vi "LoadDataSPC130.vi"(5 "Path":refnum<vi>) -> (0 "gap photons":u32, 1 "invalid photons":u32, 2 "total":u32)   [LabVIEW 2009]
panel:
  out "% done":dbl(slide) scale=0.0..100.0
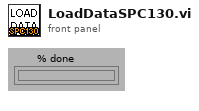
[diagram p1: front panel]
types:
  T1 = enum16{"Display", "change", "Get", "Set", "Set Ken"}
  T2 = typedef "FIFOSettings_BH.ctt" = cluster{"Measurement":cluster{"Binning (ms)":sgl, "External Trigger Condition":u16, "Stop Condition:":u16, "Stop Count":dbl, "Buffer Size (Photons)":u16, "No of Channels":u16, "Ext Latch Delay":i16}, "ADC":cluster{"Module":u16, "ADC Resolution":i32, "Dither Range":i16, "Count Increment":i16, "Macro Time Clock":i16}, "SYNC":cluster{"SYNC ZC Level (mV)":sgl, "SYNC Freq Divider":i16, "SYNC Holdoff (ns)":sgl, "SYNC Threshold (mV)":sgl}, "TAC":cluster{"TAC Range (ns)":sgl, "TAC Gain":i16, "TAC Offset (%)":sgl, "TAC Limit Low (%)":sgl, "TAC Limit High (%)":sgl}, "CFD":cluster{"CFD Limit Low (mV)":sgl, "CFD Limit High (mV)":sgl, "CFD ZC Level (mV)":sgl, "CFD Holdoff (ns)":sgl}}
  T3 = cluster{"router channels":u8[], "macro times":dbl[], "micro times":u16[], "invalid times":dbl[], "gap times":dbl[]}
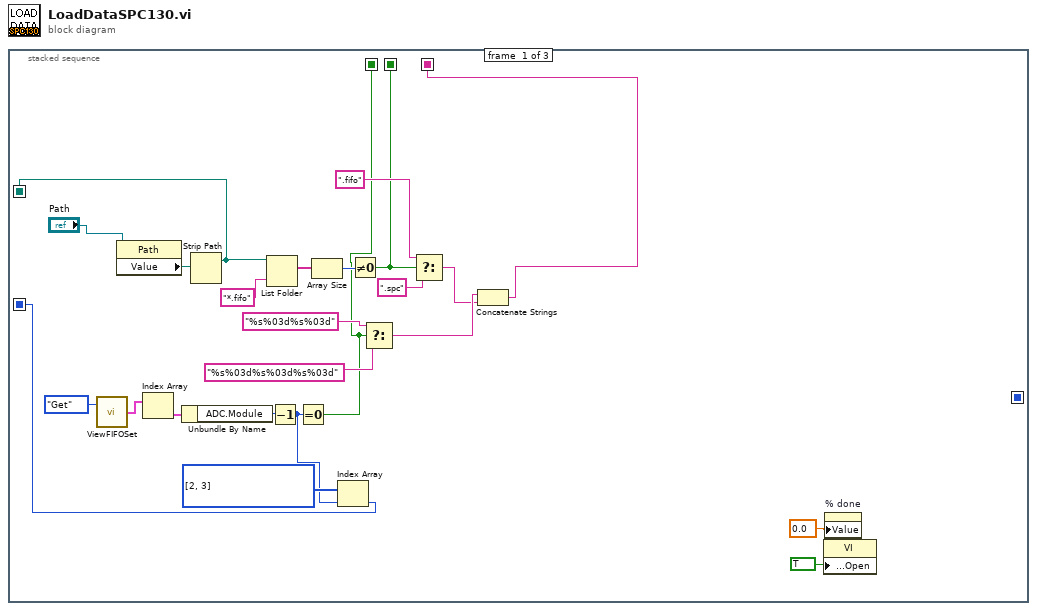
[diagram p0: block diagram]
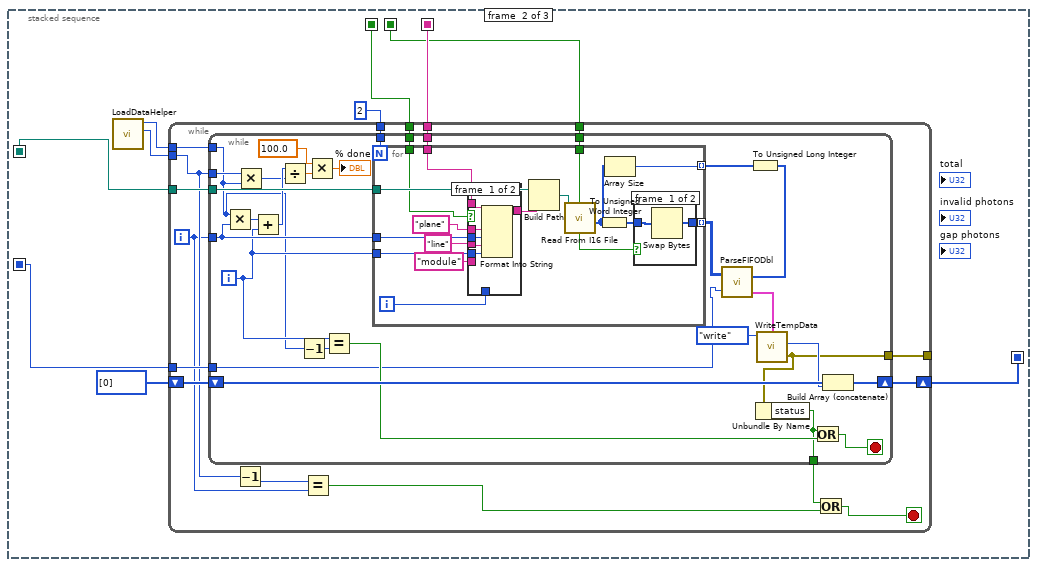
[diagram p2: hidden frame]
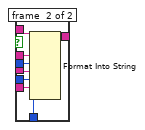
[diagram p3: hidden frame]
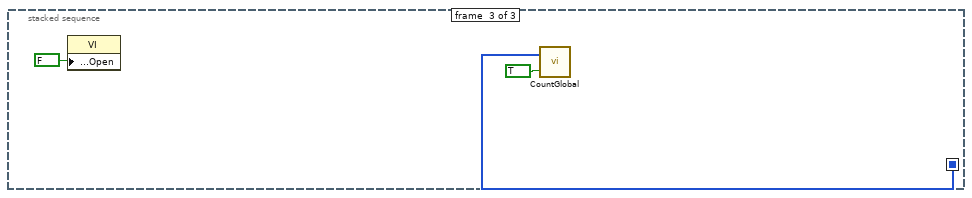
[diagram p5: hidden frame]
diagram:
  n1 = stacked-sequence {
    seq-local: [_ w33 _] -> [_ _ w115]
    seq-local: [w16 _ _] -> [_ w29 _]
    seq-local: [w15 _ _] -> [_ w25 _]
    seq-local: [w6 _ _] -> [_ w28 _]
    seq-local: [w2 _ _] -> [_ w27 _]
    seq-local: [w1 _ _] -> [_ w26 _]
    frame #0 {
      w4 = u16[] [2, 3] items=["SPC 630 - 32 bit", "SPC 630 - 48 bit", "SPC 830 - 32 bit", "SPC 130 - 32 bit", ""]
      n2 = call "ViewFIFOSet.vi"("Enum"=T1."Get") -> ("FIFO Settings (Array)"=w12:T2[])  [unwired: 1 in]
      n3 = property on="Property Node" class="Path"(reference="Path") -> ("Value"=w22:path)  [unwired: 1 in, 2 out]
      n4 = Index Array(array=w12) -> (element=w13:T2)  [unwired: 1 in]
      n5 = Unbundle By Name(w13) -> ("ADC.Module"=w11:u16)
      n6 = Strip Path(path=w22) -> (stripped path=w16:path)  [unwired: 1 out]
      n7 = List Folder(path=w16, pattern="*.fifo") -> (filenames=w20:string[])  [unwired: 2 in, 3 out]
      n8 = Decrement(x=w11) -> (x-1=w3:u16)
      n9 = Equal To 0?(x=w3) -> (x = 0?=w1:bool)
      n10 = Array Size(array=w20) -> (size(s)=w19:i32)
      n11 = Index Array(array=w4, index=w3) -> (element=w2:u16)
      n12 = Not Equal To 0?(x=w19) -> (x != 0?=w15:bool)
      n13 = Select(t="%s%03d%s%03d" ("format string"), s=w1, f="%s%03d%s%03d%s%03d" ("format string")) -> (s? t:f=w8:string)
      n14 = Select(t=".fifo" ("format string"), s=w15, f=".spc" ("format string")) -> (s? t:f=w7:string)
      n15 = Concatenate Strings(w8, w7) -> (w6:string)
      n16 = property class="VI"("Front Panel Window:Open"=TRUE) -> ()  [unwired: 2 in, 2 out]
      n17 = property on="% done" class="Slide (strict)"("Value"=0.0 ("% done")) -> ()  [unwired: 2 in, 2 out]
    }
    frame #1 {
      n18 = call "LoadDataHelper.vi"() -> ("planes"=w30:u32, "lines"=w32:u32)  [unwired: 7 in, 3 out]
      n19 = while {
        tunnel: w32 -> [w45]
        tunnel: w29 -> [w50]
        tunnel: w27 -> [w49]
        shift-right: [w47] -> w33
        shift-left: i32[] [0] -> [w48]
        tunnel: 2 -> [w46]
        tunnel: w30 -> [w39]
        tunnel: [w44] -> _
        tunnel: w28 -> [w37]
        tunnel: w25 -> [w36]
        tunnel: w26 -> [w35]
        i -> [w38]
        stop <- w41 stop-if-true
        n20 = while {
          tunnel: w50 -> [w79]
          tunnel: w38 -> [w73]
          tunnel: w49 -> [w53]
          shift-right: [w77] -> w47
          shift-left: w48 -> [w78]
          tunnel: w39 -> [w70]
          tunnel: w46 -> [w68]
          tunnel: w45 -> [w58]
          tunnel: [w63] -> w44
          tunnel: [w61] -> w43
          tunnel: w37 -> [w57]
          tunnel: w36 -> [w56]
          tunnel: w35 -> [w55]
          i -> [w64]
          stop <- w60 stop-if-true
          n21 = Multiply(x=w58, y=w73) -> (x*y=w71:u32)
          n22 = Multiply(x=w70, y=w58) -> (x*y=w69:u32)
          n23 = Add(x=w71, y=w64) -> (x+y=w72:u32)
          n24 = Divide(x=w72, y=w69) -> (x/y=w76:dbl)
          n25 = Decrement(x=w58) -> (x-1=w59:u32)
          n26 = Multiply(x=100.0, y=w76) -> (x*y=→"% done":dbl)
          n27 = Equal?(x=w64, y=w59) -> (x = y?=w62:bool)
          n28 = for {
            N: w68 -> [_]
            tunnel: w79 -> [w95]
            tunnel: w64 -> [w90]
            tunnel: w73 -> [w89]
            tunnel: [w83] -> w54 mode=indexing
            tunnel: [w85] -> w67 mode=indexing
            tunnel: w57 -> [w82]
            tunnel: w56 -> [w81]
            tunnel: w55 -> [w80]
            i -> [w84]
            n29 = case shown="True" w80 {
              tunnel: "plane" -> [w101 w109]
              tunnel: "line" -> [w100 w108]
              tunnel: [w99 w107] -> w92
              tunnel: w90 -> [w98 w106]
              tunnel: w89 -> [w97 w105]
              tunnel: "module" -> [_ w104]
              tunnel: w84 -> [_ w103]
              tunnel: w82 -> [w96 w102]
              frame #0 {
                n30 = Format Into String(format string=w96, w101, w97, w100, w98) -> (resulting string=w99:string)  [unwired: 2 in, 1 out]
              }
              frame #1 {
                n31 = Format Into String(format string=w102, w109, w105, w108, w106, w104, w103) -> (resulting string=w107:string)  [unwired: 2 in, 1 out]
              }
            }
            n32 = Build Path(base path=w95, name or relative path=w92) -> (appended path=w91:path)
            n33 = call "Read From I16 File.vi"("file path (dialog if empty)"=w91) -> ("1D array"=w86:i16[])  [unwired: 6 in, 4 out]
            n34 = To Unsigned Word Integer(number=w86) -> (unsigned 16bit integer=w87:u16[])
            n35 = Array Size(array=w86) -> (size(s)=w85:i32)
            n36 = case shown="True" w81 {
              tunnel: w87 -> [w111 w112]
              tunnel: [w110 w112] -> w83
              frame #0 {
                n37 = Swap Bytes(anything=w111) -> (byte swapped=w110:u16[])
              }
              frame #1 {
              }
            }
          }
          n38 = To Unsigned Long Integer(number=w67) -> (unsigned 32bit integer=w51:u32[])
          n39 = call "ParseFIFODbl.vi"("photoncount"=w51, "SPC Format"=w53, "FIFO rawdata"=w54) -> ("rawdata"=w52:T3)
          n40 = call "WriteTempData.vi"("rawdata"=w52, "Enum"=enum16{"create new", "write", "close"}."write") -> ("offset"=w65:i32, "error out"=w63:errorcluster)  [unwired: 3 in]
          n41 = Unbundle By Name(w63) -> ("status"=w61:bool)
          n42 = Or(x=w61, y=w62) -> (x .or. y?=w60:bool)
          n43 = Build Array (concatenate)(w78, w65) -> (w77:i32[])
        }
        n44 = Decrement(x=w39) -> (x-1=w40:u32)
        n45 = Equal?(x=w40, y=w38) -> (x = y?=w42:bool)
        n46 = Or(x=w43, y=w42) -> (x .or. y?=w41:bool)
      }
    }
    frame #2 {
      n47 = property class="VI"("Front Panel Window:Open"=FALSE) -> ()  [unwired: 2 in, 2 out]
      n48 = call "CountGlobal.vi"("changed?"=TRUE, "count"=w115) -> ()  [unwired: 1 in, 1 out]
    }
  }
